vi "get data interface information.vi"(11 "fixed channel runtime in":refnum<class "fixed channel runtime.lvclass">) -> (2 "data type defs":T1, 3 "fixed channel runtime out":refnum<class "fixed channel runtime.lvclass">)   [LabVIEW 2013, in "fixed channel runtime.lvclass"]
uses:
  fixed channel runtime.lvclass
  data cluster type definition.ctl
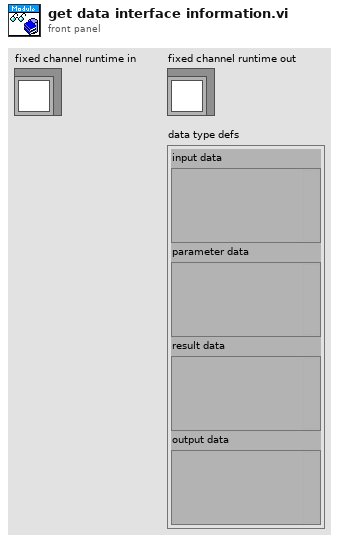
[diagram p1: front panel]
types:
  T1 = typedef "fixed channel runtime.lvclass/data cluster type definition.ctl" = cluster{"input data":variant, "parameter data":variant, "result data":variant, "output data":variant}
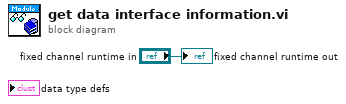
[diagram p0: block diagram]
diagram:
  "fixed channel runtime out" <- "fixed channel runtime in"
